vi "STOP.vi"(8 "error in (no error)":errorcluster, 11 "Inst.Xeryon-Rotator in":refnum<class "Inst.Xeryon-Rotator.lvclass">) -> (0 "error out":errorcluster, 3 "Inst.Xeryon-Rotator out":refnum<class "Inst.Xeryon-Rotator.lvclass">)   [LabVIEW 2019, in "Inst.Xeryon-Rotator.lvclass"]
uses:
  Inst.Xeryon-Rotator.lvclass
  drivers/Class/Controller/Controller.lvclass
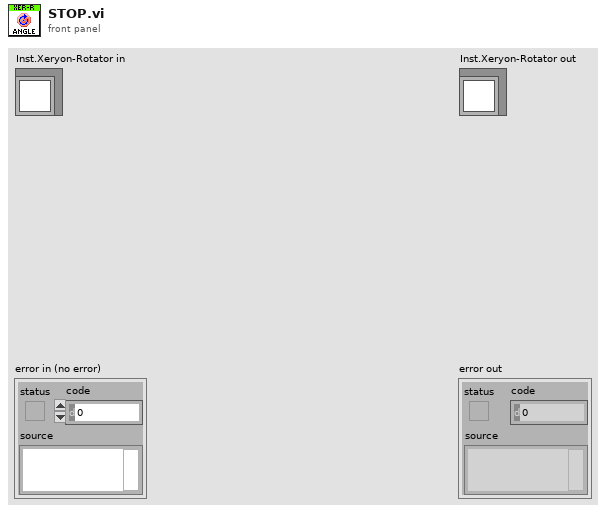
[diagram p1: front panel]
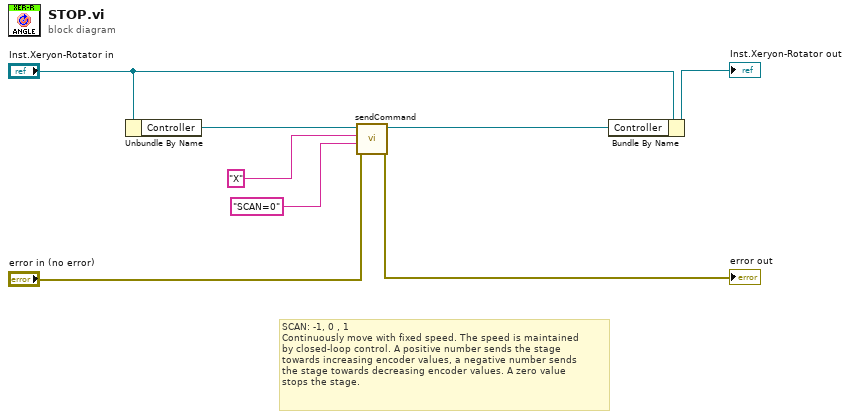
[diagram p0: block diagram]
diagram:
  # "SCAN: -1, 0 , 1\nContinuously move with fixed speed. The speed is maintained\nby closed-loop control. A positive number sends the stage\ntowards increasing encoder values, a negative number sends\nthe stage towards decreasing encoder values. A zero value\nstops the stage."
  n1 = Unbundle By Name("Inst.Xeryon-Rotator in") -> ("Controller"=w6:refnum<class "Controller.lvclass">)
  n2 = call-dynamic "sendCommand.vi"("error in (no error)"="error in (no error)", "Command"="SCAN=0", "Axis Letter"="X", "Controller in"=w6) -> ("error out"=→"error out":errorcluster, "Controller out"=w4:refnum<class "Controller.lvclass">)  [unwired: 6 in]
  n3 = Bundle By Name(cluster="Inst.Xeryon-Rotator in", "Controller"=w4) -> (→"Inst.Xeryon-Rotator out":refnum<class "Inst.Xeryon-Rotator.lvclass">)
